vi "Response - Set Body.vi"() -> (3 "Unit Test Framework Results":T1)   [LabVIEW 2017, in "Response.lvclass"]
doc: "Use this template to create a user-defined test VI. Define your test requirements and wire the results to the <b>Result (Test)</b> control. Do not modify the <b>Unit Test Framework Results</b> indicator."
uses:
  Response.lvclass
  <vilib>/utf/common/utf_test_comparison_operators.ctl
  <vilib>/utf/NI_UnitTestFramework.lvlib
  <vilib>/utf/common/utf_test_result.ctl
  <vilib>/utf/common/utf_test_result_failure.ctl
  <vilib>/utf/common/utf_test_result_troll.ctl
  <vilib>/utf/common/utf_vi_tag.ctl
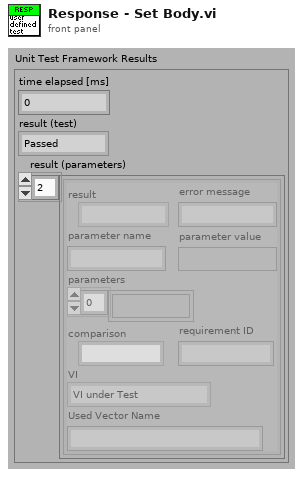
[diagram p1: front panel]
types:
  T1 = typedef "NI_UnitTestFramework.lvlib/utf_test_result_troll.ctl" = cluster{"time elapsed [ms]":u32, "result (test)":T2, "result (parameters)":T3[]}
  T2 = typedef "NI_UnitTestFramework.lvlib/utf_test_result.ctl" = enum16{"Passed", "Failed", "Error", "Skipped", "Not Processed"}
  T3 = typedef "NI_UnitTestFramework.lvlib/utf_test_result_failure.ctl" = cluster{"result":T2, "error message":string, "parameter name":string, "parameter value":variant, "parameters":variant[], "comparison":T4, "requirement ID":string, "VI":T5, "Used Vector Name":string}
  T4 = typedef "NI_UnitTestFramework.lvlib/utf_test_comparison_operators.ctl" = enum16{"=", "!=", ">", ">=", "<", "<=", "range", "symmetric tolerance", "asymmetric tolerance", "string contains", "string not contain", "array size", "string length", "array range", "by element", "array range (limit array)", "user-defined", "array contains", "array not contain", "vector length", "= (elm)", "!= (elm)", "= (case insensitive)", "!= (case insensitive)"}
  T5 = typedef "NI_UnitTestFramework.lvlib/utf_vi_tag.ctl" = enum16{"Setup VI", "VI under Test", "Teardown VI"}
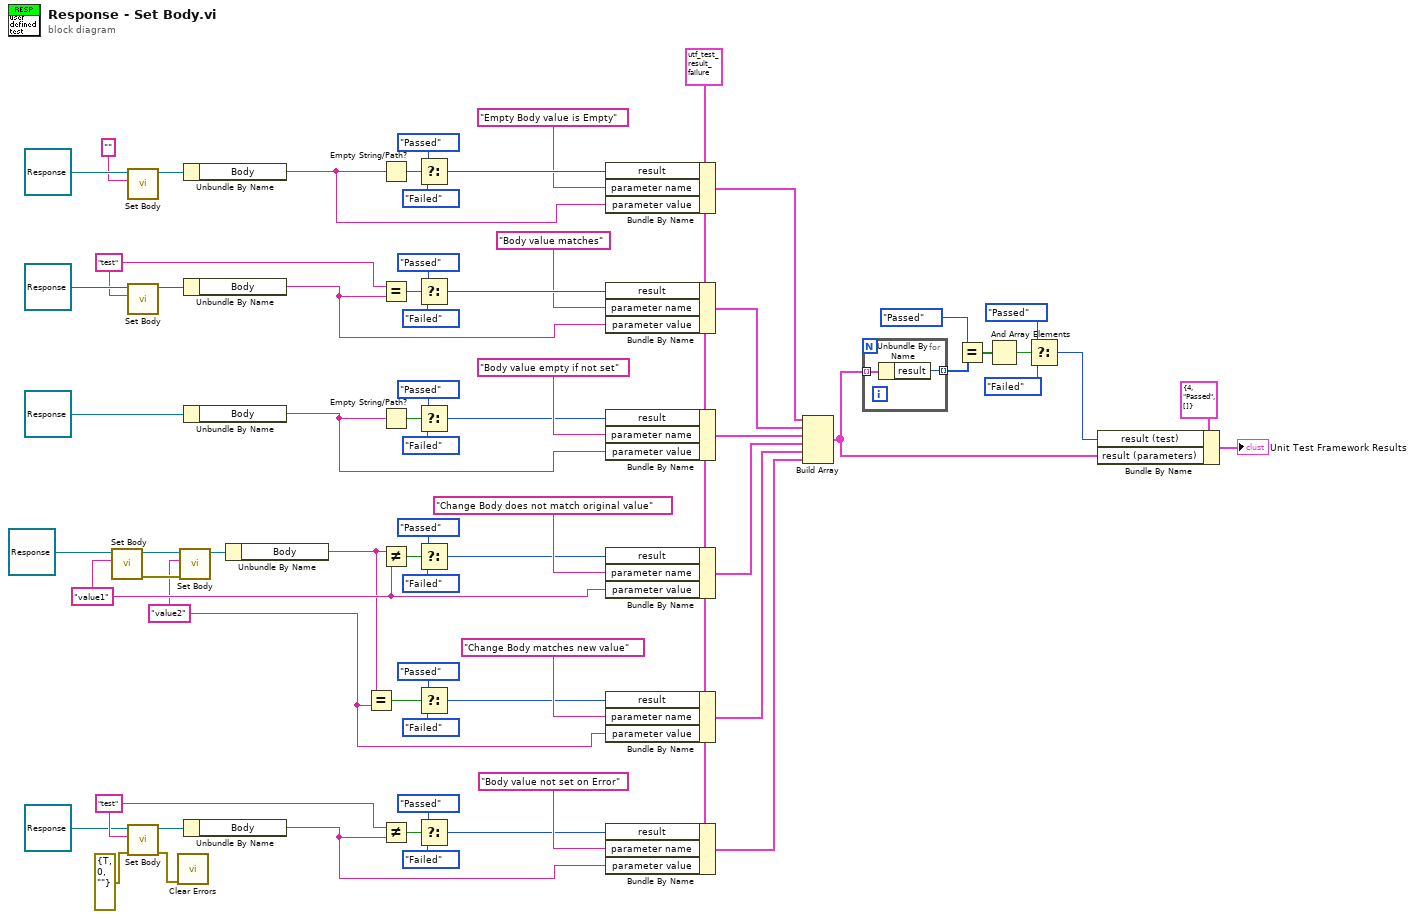
[diagram p0: block diagram]
diagram:
  w12 = "test" ("parameter name")
  w14 = "value2" ("parameter name")
  w16 = "value1" ("parameter name")
  w29 = "test" ("parameter name")
  w4 = T3 {"result"=enum."Not Processed", "error message"="", "parameter name"="", "parameter value"=variant, "parameters"=[], "comparison"=enum."=", "requirement ID"="", "VI"=enum."VI under Test", "Used Vector Name"=""} ("Unit Test Framework - result (parameters)")
  n1 = call "Set Body.vi"("Header"=w16, "Response in"=refnum<class "Response.lvclass"> refnum) -> ("error out"=w46:errorcluster, "Response out"=w40:refnum<class "Response.lvclass">)  [unwired: 8 in]
  n2 = call "Set Body.vi"("Header"="" ("parameter name"), "Response in"=refnum<class "Response.lvclass"> refnum) -> ("Response out"=w31:refnum<class "Response.lvclass">)  [unwired: 8 in, 1 out]
  n3 = call "Set Body.vi"("Header"=w29, "Response in"=refnum<class "Response.lvclass"> refnum) -> ("Response out"=w30:refnum<class "Response.lvclass">)  [unwired: 8 in, 1 out]
  n4 = call "Set Body.vi"("error in (no error)"=errorcluster {"status"=TRUE, "code"=0, "source"=""}, "Header"=w12, "Response in"=refnum<class "Response.lvclass"> refnum) -> ("error out"=w1:errorcluster, "Response out"=w11:refnum<class "Response.lvclass">)  [unwired: 7 in]
  n5 = call <vilib>:"Clear Errors.vi"("error in (no error)"=w1) -> ()  [unwired: 5 in, 2 out]
  n6 = call "Set Body.vi"("error in (no error)"=w46, "Header"=w14, "Response in"=w40) -> ("Response out"=w17:refnum<class "Response.lvclass">)  [unwired: 7 in, 1 out]
  n7 = Unbundle By Name(w31) -> ("Body"=w19:string)
  n8 = Unbundle By Name(w30) -> ("Body"=w20:string)
  n9 = Unbundle By Name(refnum<class "Response.lvclass"> refnum ("Response in")) -> ("Body"=w21:string)
  n10 = Unbundle By Name(w11) -> ("Body"=w13:string)
  n11 = Unbundle By Name(w17) -> ("Body"=w15:string)
  n12 = Equal?(x=w15, y=w14) -> (x = y?=w37:bool)
  n13 = Empty String/Path?(string/path=w19) -> (empty?=w68:bool)
  n14 = Equal?(x=w29, y=w20) -> (x = y?=w53:bool)
  n15 = Empty String/Path?(string/path=w21) -> (empty?=w26:bool)
  n16 = Not Equal?(x=w15, y=w16) -> (x != y?=w44:bool)
  n17 = Not Equal?(x=w12, y=w13) -> (x != y?=w8:bool)
  n18 = Select(t=utf_test_result."Passed" ("result"), s=w68, f=utf_test_result."Failed" ("result")) -> (s? t:f=w67:T2)
  n19 = Select(t=utf_test_result."Passed" ("result"), s=w53, f=utf_test_result."Failed" ("result")) -> (s? t:f=w54:T2)
  n20 = Select(t=utf_test_result."Passed" ("result"), s=w26, f=utf_test_result."Failed" ("result")) -> (s? t:f=w25:T2)
  n21 = Select(t=utf_test_result."Passed" ("result"), s=w44, f=utf_test_result."Failed" ("result")) -> (s? t:f=w43:T2)
  n22 = Select(t=utf_test_result."Passed" ("result"), s=w37, f=utf_test_result."Failed" ("result")) -> (s? t:f=w35:T2)
  n23 = Select(t=utf_test_result."Passed" ("result"), s=w8, f=utf_test_result."Failed" ("result")) -> (s? t:f=w7:T2)
  n24 = Bundle By Name(cluster=w4, "result"=w67, "parameter name"="Empty Body value is Empty", "parameter value"=w19) -> (w38:T3)
  n25 = Bundle By Name(cluster=w4, "result"=w54, "parameter name"="Body value matches", "parameter value"=w20) -> (w28:T3)
  n26 = Bundle By Name(cluster=w4, "result"=w25, "parameter name"="Body value empty if not set", "parameter value"=w21) -> (w18:T3)
  n27 = Bundle By Name(cluster=w4, "result"=w43, "parameter name"="Change Body does not match original value", "parameter value"=w16) -> (w39:T3)
  n28 = Bundle By Name(cluster=w4, "result"=w35, "parameter name"="Change Body matches new value", "parameter value"=w14) -> (w32:T3)
  n29 = Bundle By Name(cluster=w4, "result"=w7, "parameter name"="Body value not set on Error", "parameter value"=w13) -> (w3:T3)
  n30 = Build Array(w38, w28, w18, w39, w32, w3) -> (w64:T3[])
  n31 = for {
    tunnel: w64 -> [w72] mode=indexing
    tunnel: [w71] -> w63 mode=indexing
    n32 = Unbundle By Name(w72) -> ("result"=w71:T2)
  }
  n33 = Equal?(x=utf_test_result."Passed" ("result"), y=w63) -> (x = y?=w61:bool[])
  n34 = And Array Elements(Boolean array=w61) -> (logical AND=w60:bool)
  n35 = Select(t=utf_test_result."Passed" ("result"), s=w60, f=utf_test_result."Failed" ("result")) -> (s? t:f=w57:T2)
  n36 = Bundle By Name(cluster=T1 {"time elapsed [ms]"=4, "result (test)"=enum."Passed", "result (parameters)"=[]} ("Unit Test Framework - Result"), "result (test)"=w57, "result (parameters)"=w64) -> (→"Unit Test Framework Results":T1)
